vi "Set Data Output Format [DOF].vi"(7 "Micropulse # In":i32, 8 "error in (no error)":errorcluster, 10 "Mode":T1=enum."8-bit Mode") -> (0 "error out":errorcluster, 5 "Micropulse # Out":i32)   [LabVIEW 2026, in "MicroPulse_Driver.lvlib"]
doc: "Description:\nSeven modes are available\n<b>0</b> - Backward compatible mode for MicroPulse 4. The standard peak mode (peak count in header) of MicroPulse 4 is not supported. Only the newer peak reporting mode that supports up to 80 peaks is implemented (Peak count in the header can be accessed by utilising BAB 1 mode). Reports 8 Bit Data. Details of the command format and output messages can be found in the MicroPulse 4 Manual.\nNote in DOF 0\nTest 1 is reported as 0.\nTest 256 is reported as 0xFF\nTest 511 is reported as 0xFFE.\nThis mode is therefore of limited use as test numbers are duplicated in the output messages. It is for backward compatibility only.\n<b>1</b> - This mode is 8-bit data output mode\n<b>2</b> - This mode is 10-bit data output mode.\n<b>3</b> - This mode is 12-bit data output mode.\n<b>4</b> - This mode is 16-bit data output mode.\n<b>5</b> - This mode is 8-bit logarithmic data mode All data is output in logarithmic format except the integral part of the grass coupling message (GPL and GPH). Input parameters for commands are as per DOF3. This is intended for use with rectified data only.\n<b>6</b> - This mode is 12-bit packed data output mode. This gives a reduction of 25% in the number of bytes sent. This only affects Ascan data output, all other data and input parameters for commands are as per DOF3(12bit).\n\nNote in DOF 1 to 6:\nTest 1 is reported as 0x00.\nTest 256 is reported as 0xFF.\nTest 511 is reported as 0xFFE\n\nParameters:\n< Mode > : 0, 1, 2, 3, 4, 5, 6"
uses:
  <instrlib>/MicroPulse/MicroPulse_Driver.lvlib
  <instrlib>/MicroPulse/Public/Data/Datatypes/MP - data output format.ctl
  <instrlib>/MicroPulse/Private/MP-Registry Action-Enum.ctl
panel:
  in  "8-bit AScan Mode":bool caption="8-bit AScan mode [def: F]"
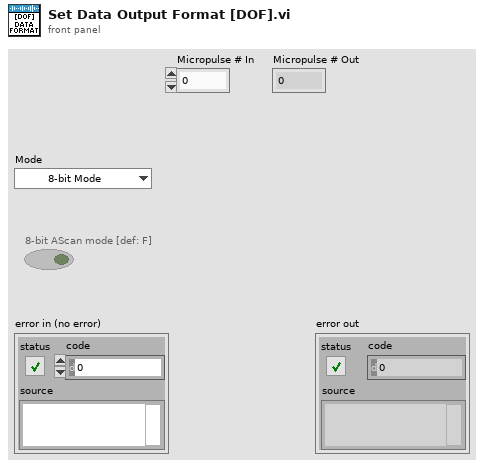
[diagram p1: front panel]
types:
  T1 = typedef "MicroPulse_Driver.lvlib/MP - data output format.ctl" = enum16{"", "8-bit Mode", "10-bit Mode", "12-bit Mode", "16-bit Mode", "8-bit Log Mode", "12-bit Packed Mode"}
  T2 = typedef "MicroPulse_Driver.lvlib/MP-Registry Action-Enum.ctl" = enum16{"Read", "Add Test", "Add Command", "Add Gate Command", "Add Encoder Command", "Clear Command  List", "Set Registry", "Set System Details", "Set DOF", "Set Velocity", "Disable Asynch Reads", "Enable Asynch Reads", "Add Connection", "Disconnect", "Shutdown"}
  T3 = typedef "MicroPulse_Driver.lvlib/TCP config.ctl" = cluster{"Connection ID":refnum<k5>, "IP address":string, "host port":u16, "OC timeout":i32, "Read timeout":i32, "Write timeout":i32}
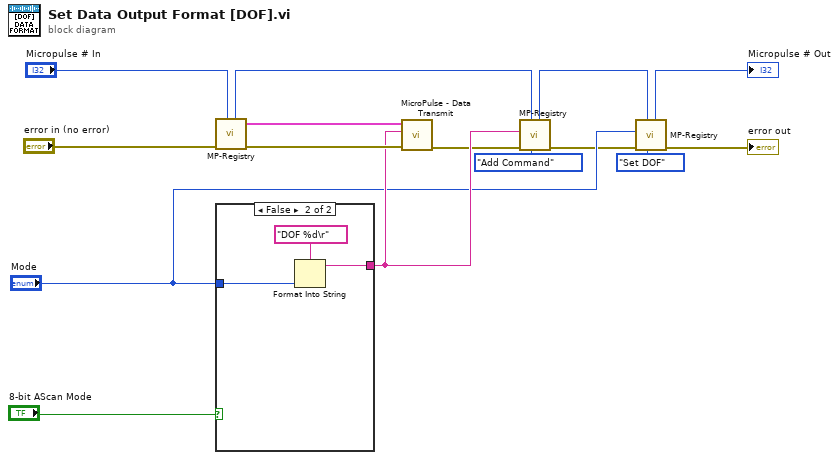
[diagram p0: block diagram]
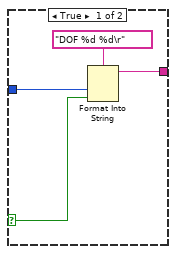
[diagram p2: hidden frame]
diagram:
  n1 = call <instrlib>:"MP-Registry.vi"("Micropulse # In"="Micropulse # In", "error in (no error)"="error in (no error)") -> ("error out"=w13:errorcluster, "TCP config"=w12:T3, "Micropulse # Out"=w8:i32)  [unwired: 6 in, 1 out]
  n2 = case shown="False" "8-bit AScan Mode" {
    selector: "8-bit AScan Mode" -> [w16 _]
    tunnel: "Mode" -> [w18 w21]
    tunnel: [w17 w20] -> w11
    frame True {
      n3 = Format Into String(format string="DOF %d %d\r", w18, w16) -> (resulting string=w17:string)  [unwired: 2 in, 1 out]
    }
    frame False {
      n4 = Format Into String(format string="DOF %d\r", w21) -> (resulting string=w20:string)  [unwired: 2 in, 1 out]
    }
  }
  n5 = call <instrlib>:"MicroPulse - Data Transmit.vi"("error in (no error)"=w13, "data"=w11, "TCP config"=w12) -> ("error out"=w9:errorcluster)  [unwired: 6 in, 2 out]
  n6 = call <instrlib>:"MP-Registry.vi"("Action"=MP-Registry_Action-Enum."Add Command", "Micropulse # In"=w8, "error in (no error)"=w9, "Data in"=w11) -> ("error out"=w2:errorcluster, "Micropulse # Out"=w4:i32)  [unwired: 4 in, 2 out]
  n7 = call <instrlib>:"MP-Registry.vi"("Action"=MP-Registry_Action-Enum."Set DOF", "Micropulse # In"=w4, "error in (no error)"=w2, "Data in"="Mode") -> ("error out"=→"error out":errorcluster, "Micropulse # Out"=→"Micropulse # Out":i32)  [unwired: 4 in, 2 out]
